vi "2d gate selection.vi"(0 "time or energy":string(combo), 1 "channel 0-4 energy in":u32[][](array[numeric]), 2 "channel 0-4 time in":u32[][](array[numeric]), 5 "Energy 2d gate":T1, 9 "Time Gate":string(combo), 11 "error in (no error)":errorcluster) -> (4 "Y name":string="channel 1", 6 "Y output array":i32[](array[numeric]), 8 "X name":string="channel 2", 10 "X output array":i32[](array[numeric]), 13 "channel 0-4 time out":u32[][](array[numeric]), 14 "channel 0-4 energy out":u32[][](array[numeric]), 15 "error out (no error)":errorcluster)   [LabVIEW 2016]
doc: "This vi is used to select which 2 signals will be used for a 2d graph. It also will pass all of the information from the \nother channels so more filtering can be applied"
uses:
  controls/energy 2d selection.ctl
panel:
  out "Channel 3 time out":u32[](array[numeric])
  out "Channel 1 time out":u32[](array[numeric])
  out "Channel 2 time out":u32[](array[numeric])
  out "Channel 0 time out":i32[](array[numeric])
  out "Channel 3 out":u32[](array[numeric])
  out "Channel 1 out":u32[](array[numeric])
  out "Channel 2 out":u32[](array[numeric])
  out "Channel 0 out":u32[](array[numeric])
  out "Channel 3 time in":u32[](array[numeric])
  out "Channel 1 time in":u32[](array[numeric])
  out "Channel 2 time in":u32[](array[numeric])
  out "Channel 0 time in":u32[](array[numeric])
  out "Channel 1":u32[](array[numeric])
  out "Channel 3":u32[](array[numeric])
  out "Channel 2":u32[](array[numeric])
  out "Channel 0":u32[](array[numeric])
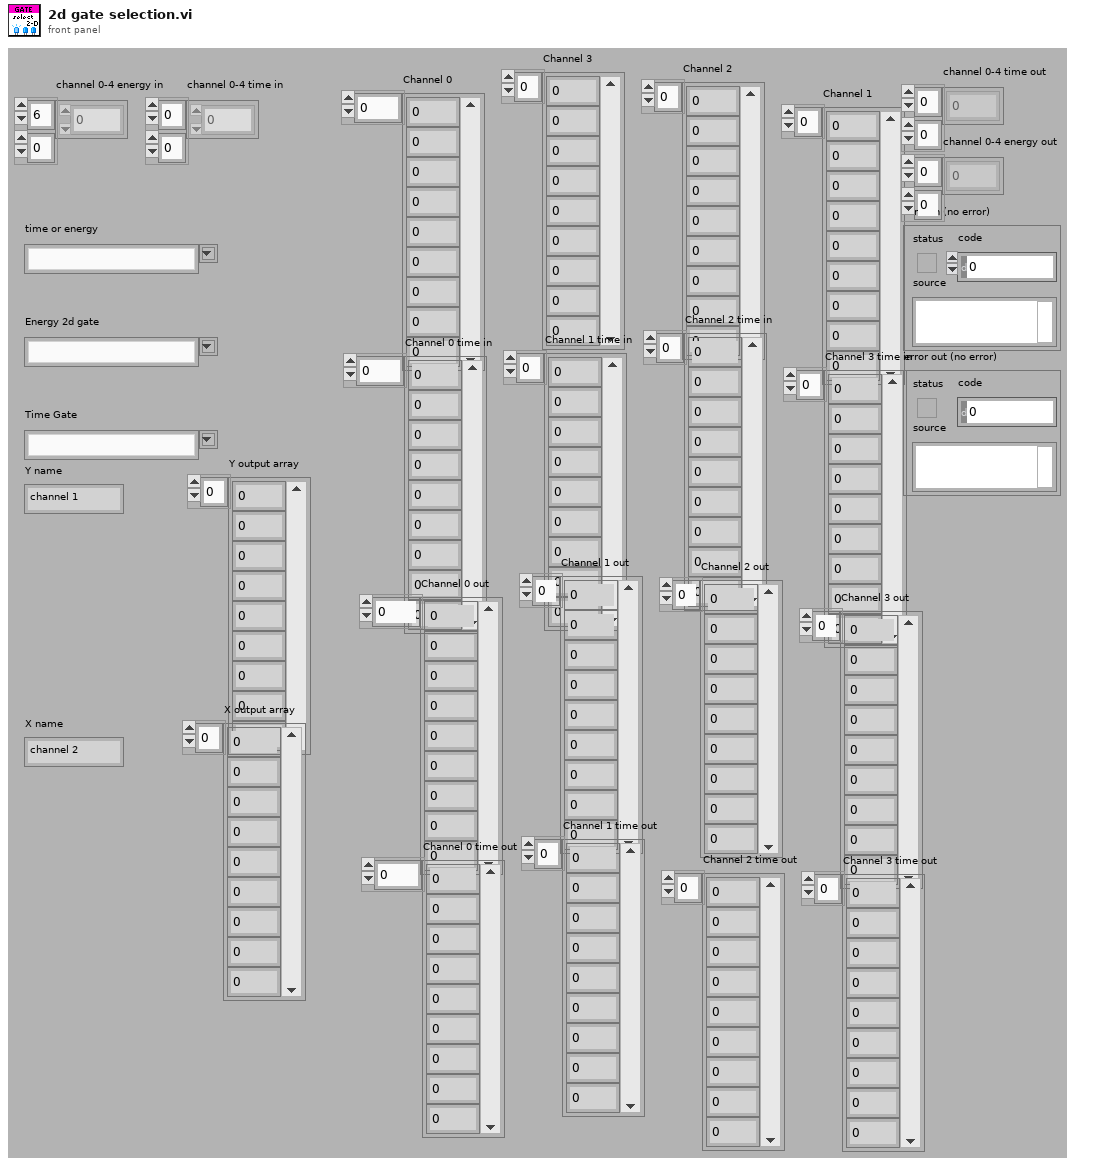
[diagram p1: front panel]
types:
  T1 = typedef "energy 2d selection.ctl" = string
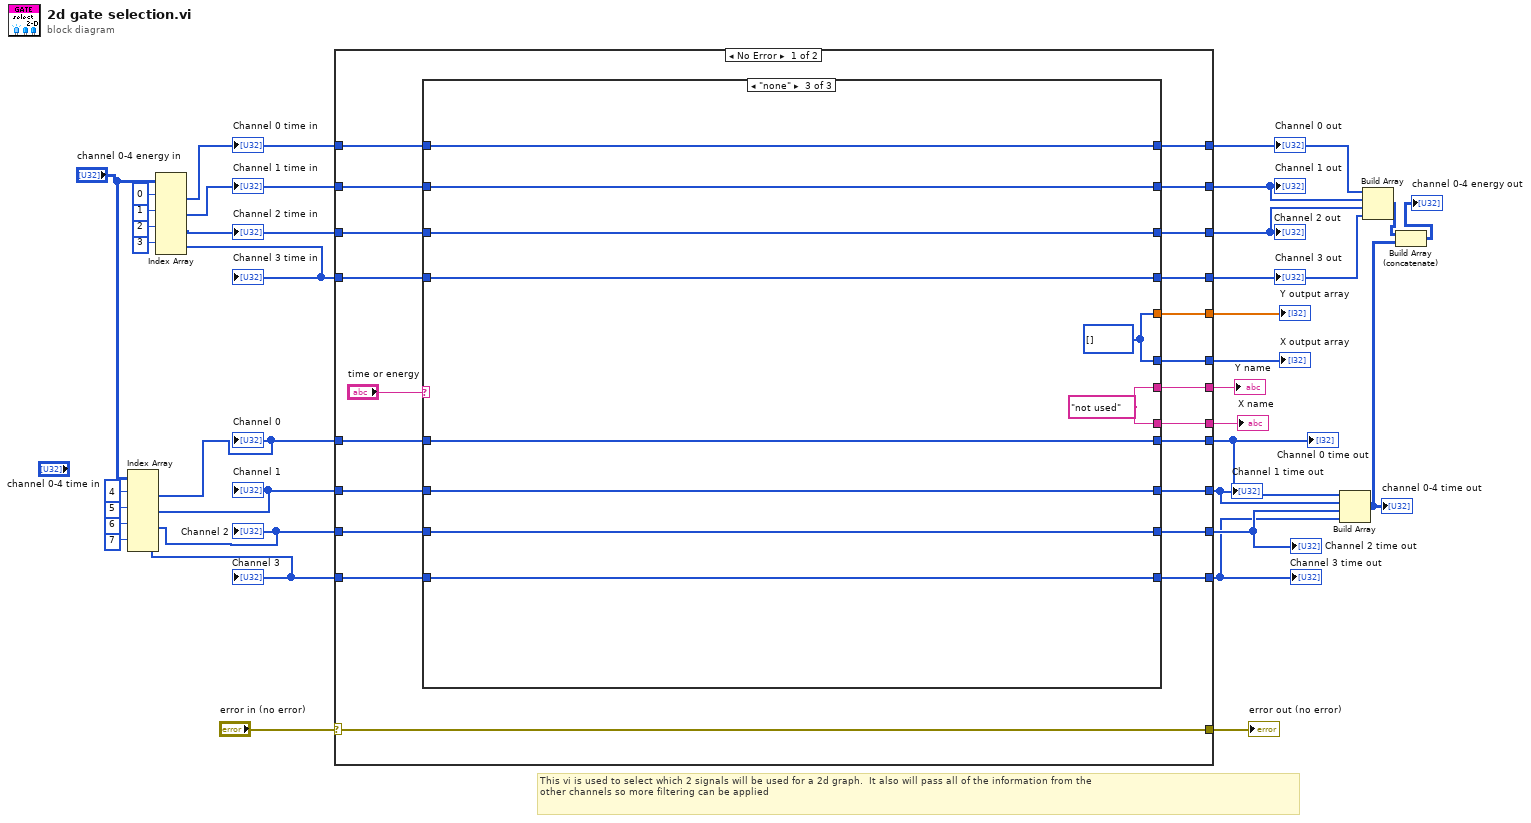
[diagram p0: block diagram]
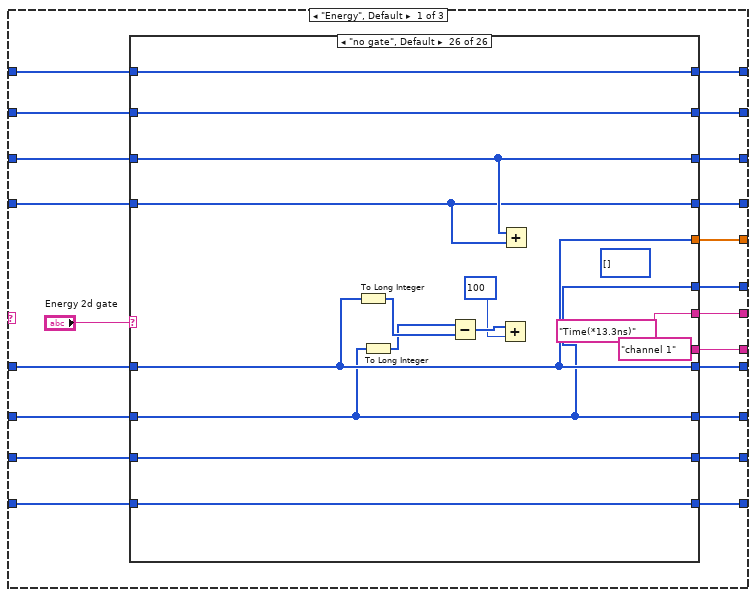
[diagram p2: hidden frame]
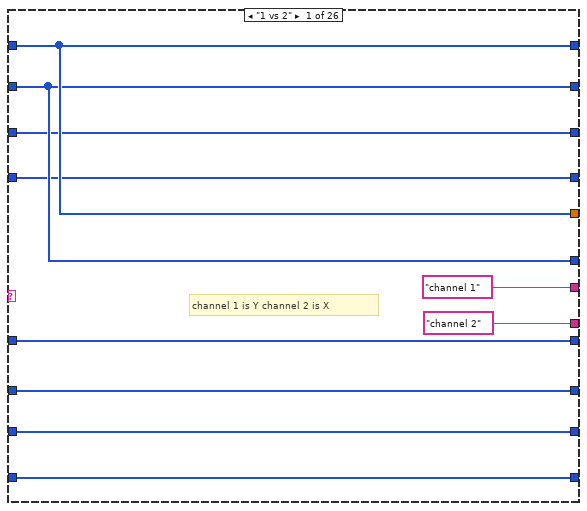
[diagram p3: hidden frame]
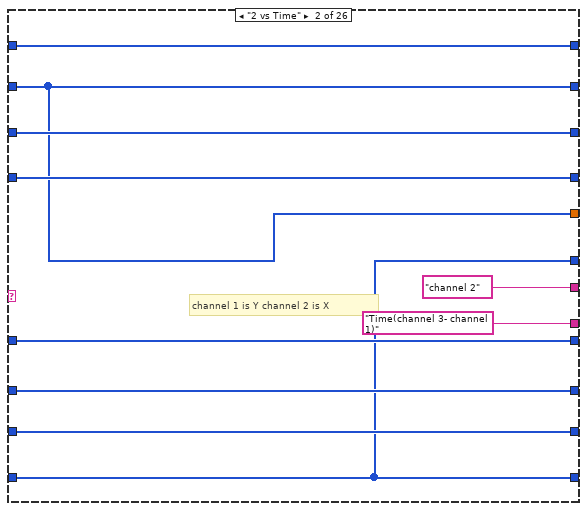
[diagram p4: hidden frame]
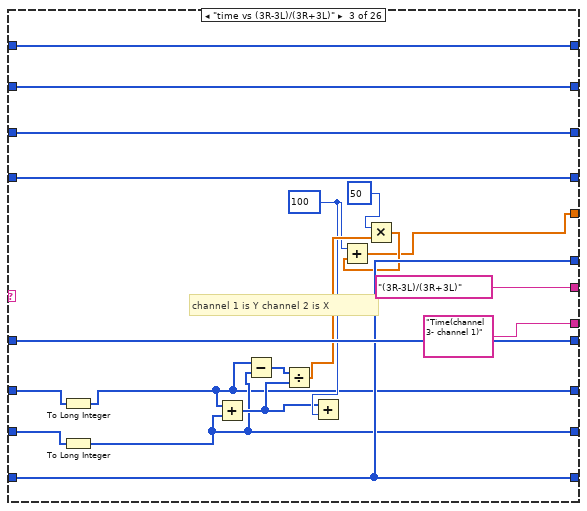
[diagram p5: hidden frame]
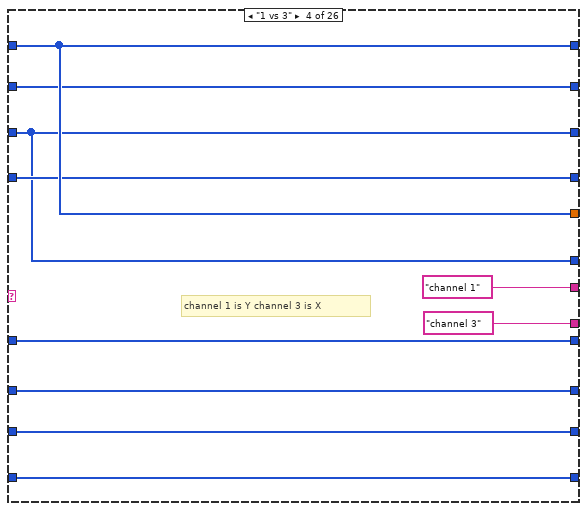
[diagram p6: hidden frame]
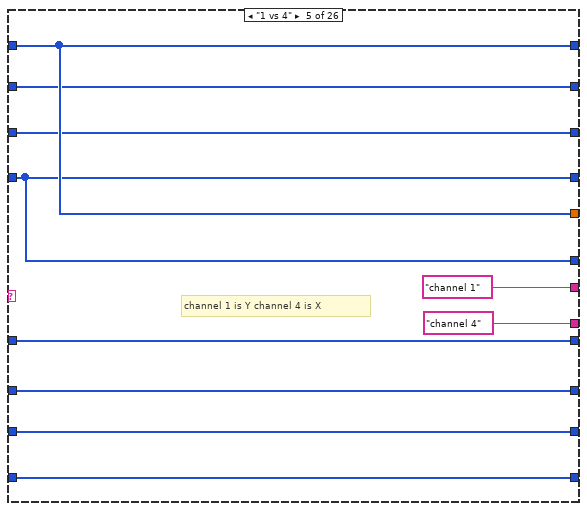
[diagram p7: hidden frame]
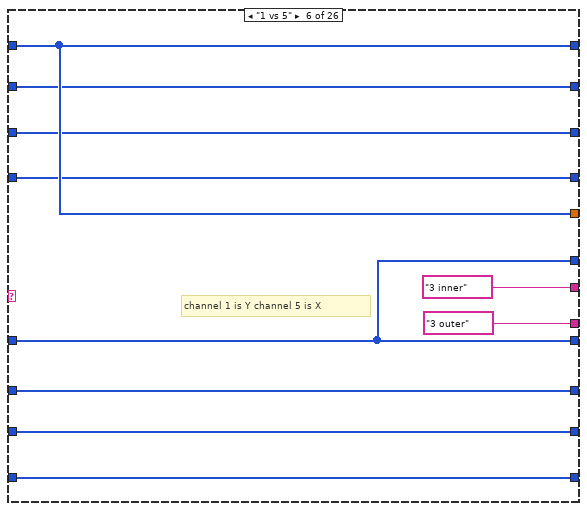
[diagram p8: hidden frame]
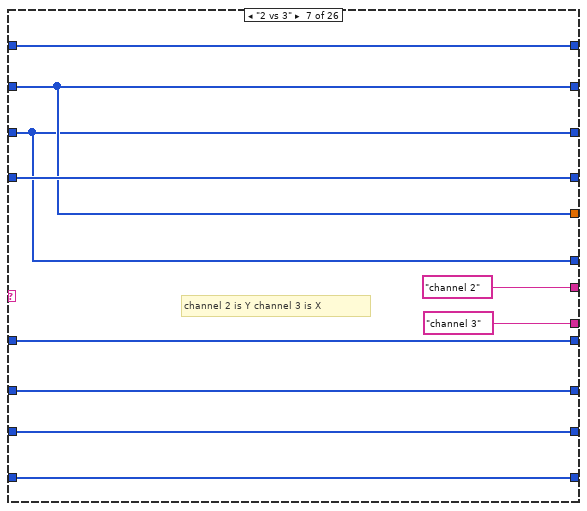
[diagram p9: hidden frame]
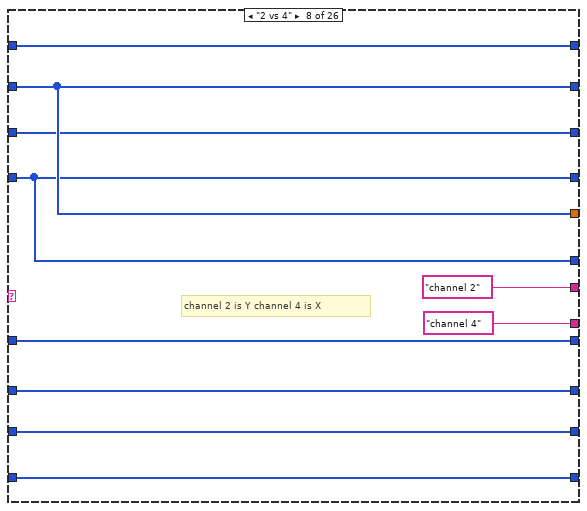
[diagram p10: hidden frame]
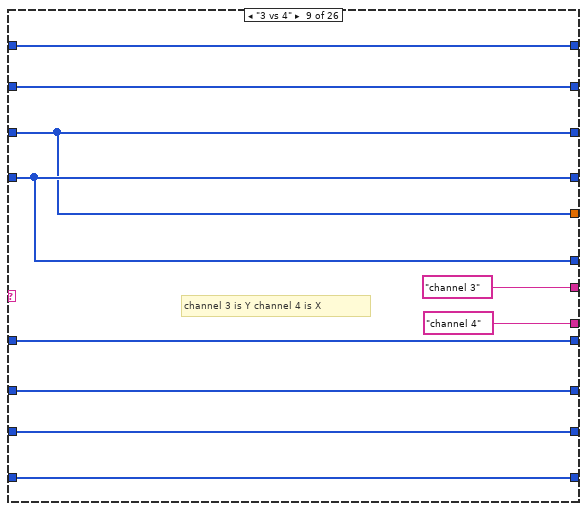
[diagram p11: hidden frame]
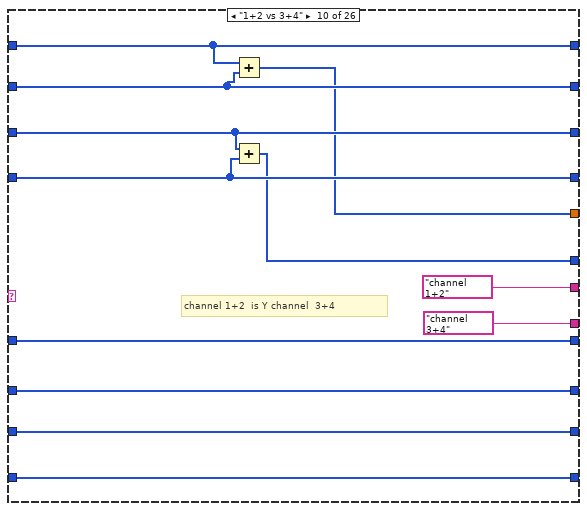
[diagram p12: hidden frame]
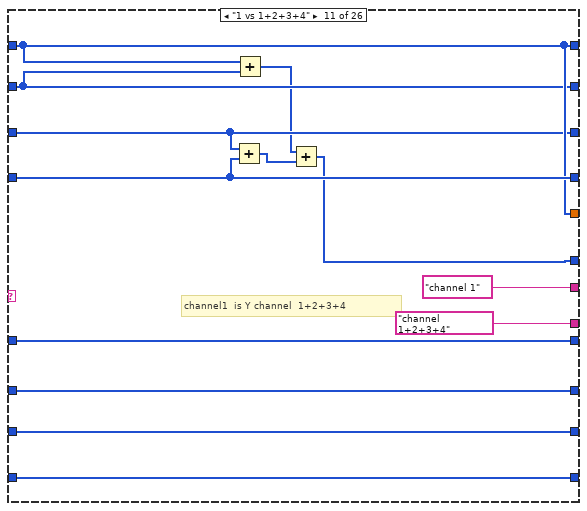
[diagram p13: hidden frame]
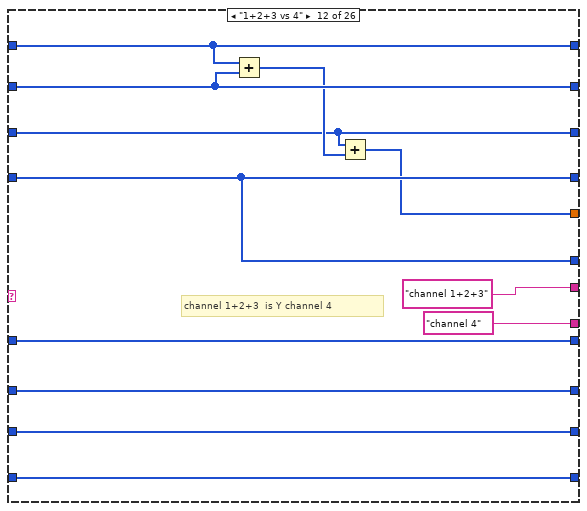
[diagram p14: hidden frame]
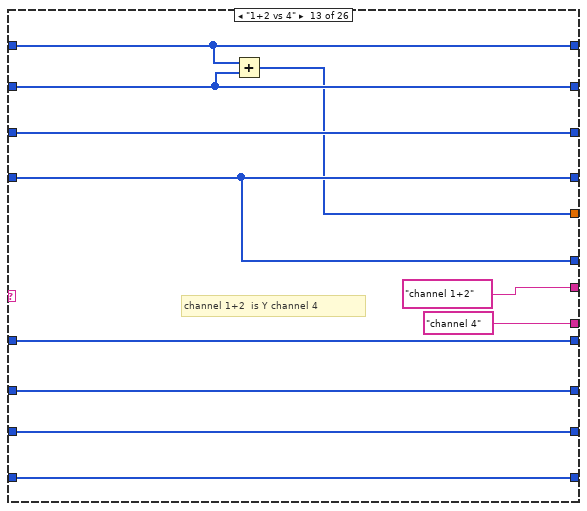
[diagram p15: hidden frame]
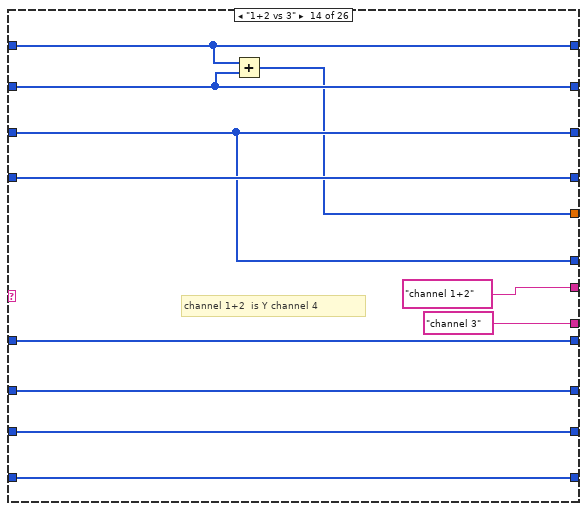
[diagram p16: hidden frame]
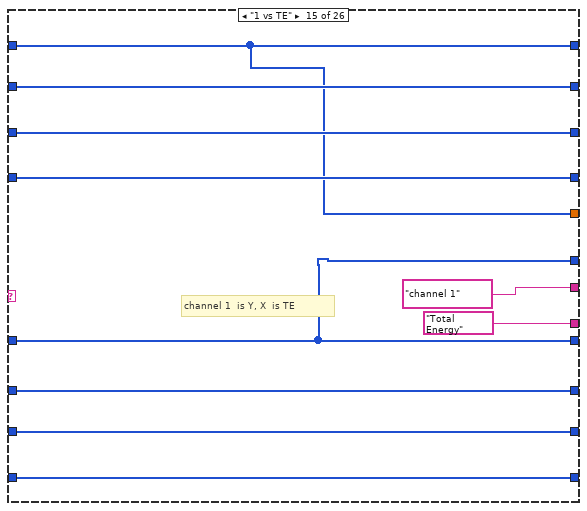
[diagram p17: hidden frame]
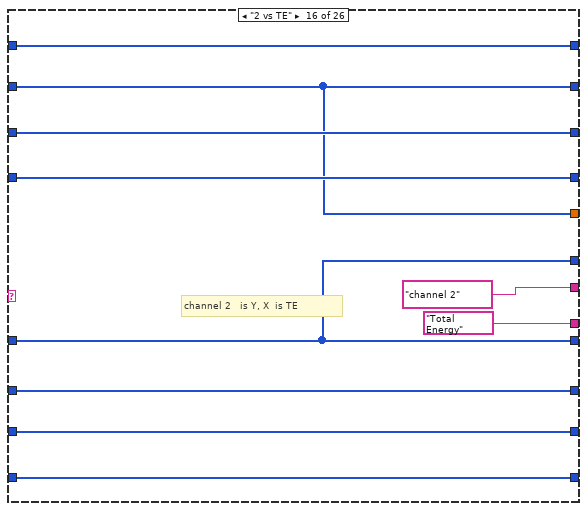
[diagram p18: hidden frame]
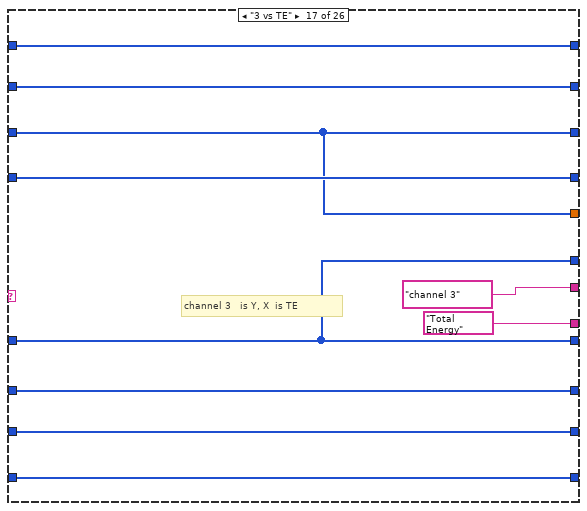
[diagram p19: hidden frame]
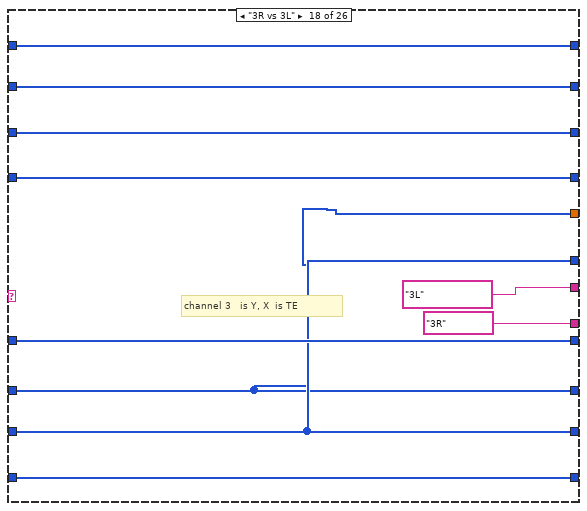
[diagram p20: hidden frame]
diagram:
  # "This vi is used to select which 2 signals will be used for a 2d graph.  It also will pass all of the information from the \nother channels so more filtering can be applied"
  n1 = Index Array(array="channel 0-4 energy in", index (row) #1=4 ("index (row)"), index (row) #2=5 ("index (row)"), index (row) #3=6 ("index (row)"), index (row) #4=7 ("index (row)")) -> (element #1=w16:u32[], element #2=w15:u32[], element #3=w14:u32[], element #4=w13:u32[])  [unwired: 4 in]
  "Channel 0" <- w16
  "Channel 2" <- w14
  "Channel 3" <- w13
  "Channel 1" <- w15
  n2 = Index Array(array="channel 0-4 energy in", index (row) #1=0 ("index (row)"), index (row) #2=1 ("index (row)"), index (row) #3=2 ("index (row)"), index (row) #4=3 ("index (row)")) -> (element #1=w20:u32[], element #2=w19:u32[], element #3=w18:u32[], element #4=w17:u32[])  [unwired: 4 in]
  "Channel 0 time in" <- w20
  "Channel 2 time in" <- w18
  "Channel 1 time in" <- w19
  "Channel 3 time in" <- w17
  n3 = case shown="No Error" "error in (no error)" {
    selector: "error in (no error)" -> [w56 w454]
    tunnel: [w56 w454] -> w34
    tunnel: w20 -> [w55 w453]
    tunnel: [w54 w453] -> w12
    tunnel: w19 -> [w53 w452]
    tunnel: [w52 w452] -> w11
    tunnel: w18 -> [w51 w451]
    tunnel: [w50 w451] -> w10
    tunnel: [w49 w450] -> w9
    tunnel: w17 -> [w48 w450]
    tunnel: w16 -> [w47 w449]
    tunnel: [w46 w449] -> w8
    tunnel: [w45 w448] -> w7
    tunnel: w15 -> [w44 w448]
    tunnel: w14 -> [w43 w447]
    tunnel: [w42 w447] -> w6
    tunnel: w13 -> [w41 w446]
    tunnel: [w40 w446] -> w5
    tunnel: [w39 w445] -> w32
    tunnel: [w38 w445] -> w31
    tunnel: [w37 w444] -> w30
    tunnel: [w36 w444] -> w29
    frame No Error {
      n4 = case shown="\"none\"" "time or energy" {
        tunnel: w55 -> [w68 w386 w443]
        tunnel: [w64 w387 w443] -> w54
        tunnel: w53 -> [w66 w384 w442]
        tunnel: [w63 w385 w442] -> w52
        tunnel: [w62 w383 w441] -> w50
        tunnel: w51 -> [w61 w382 w441]
        tunnel: [w60 w381 w440] -> w49
        tunnel: w48 -> [w59 w380 w440]
        tunnel: [w76 w379 w439] -> w46
        tunnel: w47 -> [w75 w378 w439]
        tunnel: [w74 w376 w438] -> w45
        tunnel: w44 -> [w73 w377 w438]
        tunnel: [w72 w374 w437] -> w42
        tunnel: w43 -> [w71 w375 w437]
        tunnel: [w70 w373 w436] -> w40
        tunnel: w41 -> [w69 w372 w436]
        tunnel: [w67 w369 w435] -> w39
        tunnel: [w65 w370 w435] -> w38
        tunnel: [w58 w368 w434] -> w37
        tunnel: [w57 w367 w434] -> w36
        frame "Energy", Default {
          n5 = case shown="\"no gate\", Default" "Energy 2d gate" {
            tunnel: [w87 w97 w116 w126 w136 w137 w156 w166 w176 w188 w201 w213 w224 w235 w236 w246 w257 w275 w276 w286 w296 w307 w318 w329 w340 w354] -> w76
            tunnel: w75 -> [w87 w97 w116 w126 w136 w137 w156 w166 w176 w188 w201 w213 w224 w235 w236 w246 w257 w275 w276 w286 w296 w307 w318 w329 w340 w354]
            tunnel: [w86 w96 w98 w125 w135 w146 w155 w165 w175 w187 w200 w212 w223 w234 w245 w255 w265 w266 w285 w295 w306 w317 w328 w339 w352 w353] -> w74
            tunnel: w73 -> [w86 w96 w99 w125 w135 w146 w155 w165 w175 w187 w200 w212 w223 w234 w245 w255 w265 w266 w285 w295 w306 w317 w328 w339 w352 w353]
            tunnel: [w85 w95 w100 w124 w134 w145 w154 w164 w174 w186 w199 w211 w222 w233 w244 w254 w264 w267 w284 w294 w305 w316 w327 w338 w351 w366] -> w72
            tunnel: w71 -> [w85 w95 w101 w124 w134 w145 w154 w164 w174 w186 w199 w211 w222 w233 w244 w254 w264 w267 w284 w294 w305 w316 w327 w338 w351 w366]
            tunnel: [w84 w88 w109 w123 w133 w144 w153 w163 w173 w185 w198 w210 w221 w232 w238 w247 w256 w271 w281 w291 w302 w313 w324 w335 w348 w362] -> w70
            tunnel: w69 -> [w84 w88 w109 w123 w133 w144 w153 w163 w173 w185 w198 w210 w221 w232 w238 w247 w256 w271 w281 w291 w302 w313 w324 w335 w348 w362]
            tunnel: w68 -> [w83 w94 w115 w122 w132 w143 w152 w162 w172 w182 w194 w207 w218 w229 w237 w249 w260 w270 w280 w290 w298 w311 w323 w331 w347 w355]
            tunnel: [w83 w89 w102 w122 w132 w143 w148 w159 w167 w178 w194 w202 w214 w225 w237 w248 w258 w266 w277 w286 w297 w310 w322 w334 w341 w354] -> w67
            tunnel: w66 -> [w82 w89 w110 w121 w131 w142 w148 w159 w169 w181 w193 w206 w217 w228 w241 w248 w259 w269 w279 w289 w299 w312 w319 w332 w345 w358]
            tunnel: [w82 w88 w109 w117 w127 w137 w147 w157 w168 w177 w189 w203 w215 w226 w236 w246 w257 w267 w276 w286 w296 w307 w318 w329 w340 w353] -> w65
            tunnel: [w83 w94 w115 w122 w132 w143 w152 w162 w172 w182 w194 w207 w218 w229 w237 w249 w260 w270 w280 w290 w298 w311 w323 w331 w347 w355] -> w64
            tunnel: [w82 w89 w110 w121 w131 w142 w148 w159 w169 w181 w193 w206 w217 w228 w241 w248 w259 w269 w279 w289 w299 w312 w319 w332 w345 w358] -> w63
            tunnel: [w81 w93 w114 w117 w128 w139 w147 w158 w167 w180 w192 w204 w216 w226 w239 w250 w258 w268 w278 w288 w301 w309 w320 w333 w344 w357] -> w62
            tunnel: w61 -> [w81 w93 w114 w117 w128 w139 w147 w158 w167 w180 w192 w204 w216 w226 w239 w250 w258 w268 w278 w288 w301 w309 w320 w333 w344 w357]
            tunnel: [w80 w92 w113 w120 w127 w138 w149 w157 w168 w179 w195 w203 w215 w227 w240 w251 w261 w272 w277 w287 w300 w308 w321 w330 w342 w356] -> w60
            tunnel: w59 -> [w80 w92 w113 w120 w127 w138 w149 w157 w168 w179 w195 w203 w215 w227 w240 w251 w261 w272 w277 w287 w300 w308 w321 w330 w342 w356]
            tunnel: ["channel 1" "channel 2" "(3R-3L)/(3R+3L)" "channel 1" "channel 1" "3 inner" "channel 2" "channel 2" "channel 3" "channel 1+2" "channel 1" "channel 1+2+3" "channel 1+2" "channel 1+2" "channel 1" "channel 2" "channel 3" "3L" "channel 4" "channel 5" "channel  1+2" "channel  3+4" "channel  2+3" "channel  1+4" "channel  1+2+3+4+5" "Time(*13.3ns)"] -> w58
            tunnel: ["channel 2" "Time(channel 3- channel 1)" "Time(channel 3- channel 1)" "channel 3" "channel 4" "3 outer" "channel 3" "channel 4" "channel 4" "channel 3+4" "channel 1+2+3+4" "channel 4" "channel 4" "channel 3" "Total Energy" "Total Energy" "Total Energy" "3R" "Total Energy" "Total Energy" "Total Energy" "Total Energy" "Total Energy" "Total Energy" "Total Energy" "channel 1"] -> w57
            frame "1 vs 2" {
              # "channel 1 is Y channel 2 is X"
            }
            frame "2 vs Time" {
              # "channel 1 is Y channel 2 is X"
            }
            frame "time vs (3R-3L)/(3R+3L)" {
              w104 = 100 ("Numeric")
              # "channel 1 is Y channel 2 is X"
              n6 = To Long Integer(number=w99) -> (32bit integer=w98:i32[])
              n7 = To Long Integer(number=w101) -> (32bit integer=w100:i32[])
              n8 = Add(x=w98, y=w100) -> (x+y=w103:i32[])
              n9 = Subtract(x=w98, y=w100) -> (x-y=w108:i32[])
              n10 = Divide(x=w108, y=w103) -> (x/y=w106:dbl[])
              n11 = Add(x=w103, y=w104) -> ()  [unwired: 1 out]
              n12 = Multiply(x=50 ("Numeric"), y=w106) -> (x*y=w105:dbl[])
              n13 = Add(x=w104, y=w105) -> (x+y=w102:dbl[])
            }
            frame "1 vs 3" {
              # "channel 1 is Y channel 3 is X"
            }
            frame "1 vs 4" {
              # "channel 1 is Y channel 4 is X"
            }
            frame "1 vs 5" {
              # "channel 1 is Y channel 5 is X"
            }
            frame "2 vs 3" {
              # "channel 2 is Y channel 3 is X"
            }
            frame "2 vs 4" {
              # "channel 2 is Y channel 4 is X"
            }
            frame "3 vs 4" {
              # "channel 3 is Y channel 4 is X"
            }
            frame "1+2 vs 3+4" {
              # "channel 1+2  is Y channel  3+4"
              n14 = Add(x=w182, y=w181) -> (x+y=w178:u32[])
              n15 = Add(x=w180, y=w179) -> (x+y=w177:u32[])
            }
            frame "1 vs 1+2+3+4" {
              # "channel1  is Y channel  1+2+3+4"
              n16 = Add(x=w192, y=w195) -> (x+y=w190:u32[])
              n17 = Add(x=w194, y=w193) -> (x+y=w191:u32[])
              n18 = Add(x=w191, y=w190) -> (x+y=w189:u32[])
            }
            frame "1+2+3 vs 4" {
              # "channel 1+2+3  is Y channel 4"
              n19 = Add(x=w207, y=w206) -> (x+y=w205:u32[])
              n20 = Add(x=w204, y=w205) -> (x+y=w202:u32[])
            }
            frame "1+2 vs 4" {
              # "channel 1+2  is Y channel 4"
              n21 = Add(x=w218, y=w217) -> (x+y=w214:u32[])
            }
            frame "1+2 vs 3" {
              # "channel 1+2  is Y channel 4"
              n22 = Add(x=w229, y=w228) -> (x+y=w225:u32[])
            }
            frame "1 vs TE" {
              # "channel 1  is Y, X  is TE"
            }
            frame "2 vs TE" {
              # "channel 2   is Y, X  is TE"
            }
            frame "3 vs TE" {
              # "channel 3   is Y, X  is TE"
            }
            frame "3R vs 3L" {
              # "channel 3   is Y, X  is TE"
            }
            frame "4 vs TE" {
              # "channel 4   is Y, X  is TE"
            }
            frame "5 vs TE" {
              # "channel 5   is Y, X  is TE"
            }
            frame "1+2 vs TE" {
              # "channel 1+2   is Y, X  is TE"
              n23 = Add(x=w298, y=w299) -> (x+y=w297:u32[])
            }
            frame "3+4 vs TE" {
              # "channel 3+4   is Y, X  is TE"
              n24 = Add(x=w309, y=w308) -> (x+y=w310:u32[])
            }
            frame "2+3 vs TE" {
              # "channel 2+3   is Y, X  is TE"
              n25 = Add(x=w319, y=w320) -> (x+y=w322:u32[])
            }
            frame "1+4 vs TE" {
              # "channel 1+4   is Y, X  is TE"
              n26 = Add(x=w331, y=w330) -> (x+y=w334:u32[])
            }
            frame "1+2+3+4+5 vs TE" {
              # "channel 1+4   is Y, X  is TE"
              n27 = Add(x=w347, y=w345) -> (x+y=w346:u32[])
              n28 = Add(x=w346, y=w344) -> (x+y=w343:u32[])
              n29 = Add(x=w343, y=w342) -> (x+y=w341:u32[])
            }
            frame "no gate", Default {
              (unwired) u32[] [] ("Channel 2 time in")
              n30 = To Long Integer(number=w354) -> (32bit integer=w363:i32[])
              n31 = To Long Integer(number=w353) -> (32bit integer=w361:i32[])
              n32 = Subtract(x=w361, y=w363) -> (x-y=w365:i32[])
              n33 = Add(x=w365, y=i16 100 ("Numeric")) -> ()  [unwired: 1 out]
              n34 = Add(x=w357, y=w356) -> ()  [unwired: 1 out]
            }
          }
        }
        frame "time" {
          n35 = case shown="\"4-1 vs 2-1\"" "Time Gate" {
            tunnel: [w399 w411 w423 w433] -> w387
            tunnel: w386 -> [w399 w411 w423 w433]
            tunnel: [w398 w410 w422 w432] -> w385
            tunnel: w384 -> [w398 w410 w422 w432]
            tunnel: [w397 w409 w421 w431] -> w383
            tunnel: w382 -> [w397 w409 w421 w431]
            tunnel: [w396 w408 w420 w430] -> w381
            tunnel: w380 -> [w396 w408 w420 w430]
            tunnel: [w392 w405 w417 w429] -> w379
            tunnel: w378 -> [w392 w405 w417 w429]
            tunnel: [w395 w400 w413 w428] -> w376
            tunnel: w377 -> [w395 w400 w413 w428]
            tunnel: w375 -> [w391 w404 w412 w427]
            tunnel: [w391 w404 w412 w427] -> w374
            tunnel: [w394 w407 w419 w426] -> w373
            tunnel: w372 -> [w394 w407 w419 w426]
            tunnel: [w393 w406 w418 w425] -> w370
            tunnel: [w390 w403 w416 w425] -> w369
            tunnel: ["time 3-1 " ("Y name") "time 2-1 " ("Y name") "time 2-1 " ("Y name") w424] -> w368
            tunnel: ["time 4-1 " ("Y name") "time 4-1 " ("Y name") "time 3-1 " ("Y name") w424] -> w367
            frame "4-1 vs 3-1" {
              # "time 4-1 vs 3-1"
              n36 = Subtract(x=w391, y=w392) -> (x-y=w390:u32[])
              n37 = Subtract(x=w394, y=w392) -> (x-y=w393:u32[])
            }
            frame "4-1 vs 2-1" {
              # "time 4-1 vs 2-1"
              n38 = Subtract(x=w400, y=w405) -> (x-y=w403:u32[])
              n39 = Subtract(x=w407, y=w405) -> (x-y=w406:u32[])
            }
            frame "3-1 vs 2-1" {
              # "time 3-1 vs 2-1"
              n40 = Subtract(x=w413, y=w417) -> (x-y=w416:u32[])
              n41 = Subtract(x=w412, y=w417) -> (x-y=w418:u32[])
            }
            frame "none", Default {
              w424 = "not used"
              w425 = u32[] [] ("Channel 2 time in")
            }
          }
        }
        frame "none" {
          w434 = "not used"
          w435 = u32[] [] ("Channel 2 time in")
        }
      }
    }
    frame Error {
      w444 = "error"
      w445 = u32[] [] ("Channel 2 time in")
    }
  }
  "Channel 0 out" <- w12
  "Channel 2 out" <- w10
  "Channel 1 out" <- w11
  "Channel 3 out" <- w9
  "Channel 0 time out" <- w8
  "Channel 2 time out" <- w6
  "Channel 1 time out" <- w7
  "Channel 3 time out" <- w5
  "error out (no error)" <- w34
  "Y output array" <- w32
  "X output array" <- w31
  "Y name" <- w30
  "X name" <- w29
  n42 = Build Array(w8, w7, w6, w5) -> (w4:u32[][])
  "channel 0-4 time out" <- w4
  n43 = Build Array(w12, w11, w10, w9) -> (w3:u32[][])
  n44 = Build Array (concatenate)(w3, w4) -> (→"channel 0-4 energy out":u32[][])
